vi "Queues_Create References.vi"(7 "error in":errorcluster) -> (0 "error out":errorcluster, 3 "Queue References":T1)   [LabVIEW 2014, in "QueueMaintenance.lvlib"]
doc: "Queue Reference:\n\nDefines name queue references for each of the queued state machines. This includes a custom control for both the queue data type (cluster) and a custer of all the queue refnums."
uses:
  QueueMaintenance.lvlib
  TypeDef/QSMRef_ALL.ctl
  Queue_TESTGUIUPDATE/Controls/QSM_Reference.ctl
  Queue_TESTGUIUPDATE/Controls/QSM_DataType.ctl
  Queue_TESTGUIUPDATE/Controls/QSM_RunStates.ctl
  Queue_TEST/Controls/QSM_Reference.ctl
  Queue_TEST/Controls/QSM_DataType.ctl
  Queue_TEST/Controls/QSM_RunStates.ctl
  Queue_TEST/TestQSM.lvlib
  Queue_TESTGUIUPDATE/GUIUpdateQSM.lvlib
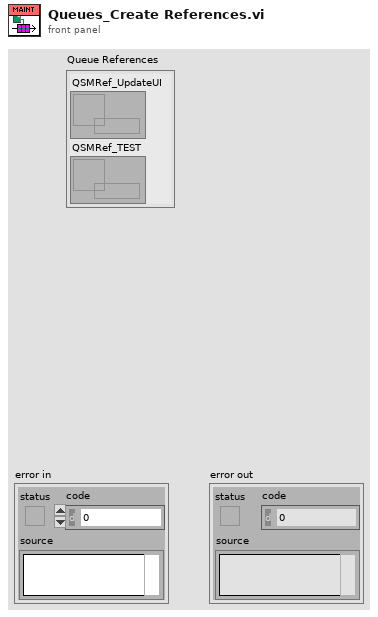
[diagram p1: front panel]
types:
  T1 = typedef "QueueMaintenance.lvlib/QSMRef_ALL.ctl" = cluster{"QSMRef_UpdateUI":T2, "QSMRef_TEST":T3}
  T2 = typedef "GUIUpdateQSM.lvlib/QSM_Reference.ctl" = refnum<queue>
  T3 = typedef "TestQSM.lvlib/QSM_Reference.ctl" = refnum<queue>
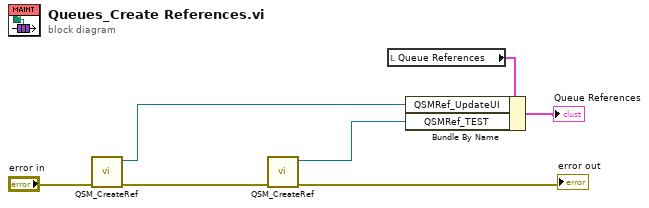
[diagram p0: block diagram]
diagram:
  n1 = call "QSM_CreateRef.vi"("error in"="error in") -> ("error out"=w2:errorcluster, "QSM_Reference out"=w1:T2)  [unwired: 9 in]
  n2 = call "QSM_CreateRef.vi"("error in"=w2) -> ("error out"=→"error out":errorcluster, "Test QSM_Reference out"=w4:T3)  [unwired: 9 in]
  n3 = local read "Queue References"() -> (w7:T1)
  n4 = Bundle By Name(cluster=w7, "QSMRef_UpdateUI"=w1, "QSMRef_TEST"=w4) -> (→"Queue References":T1)
